vi "vision angle analysis.vi"(0 "left_x":dbl, 5 "right_x":dbl, 7 "top_y":dbl, 9 "bottom_y":dbl, 11 "gyro_angle_deg":dbl) -> (4 "gyro_heading_deg":dbl, 15 "distance":dbl)   [LabVIEW 2015]
panel:
  out "other distance":dbl
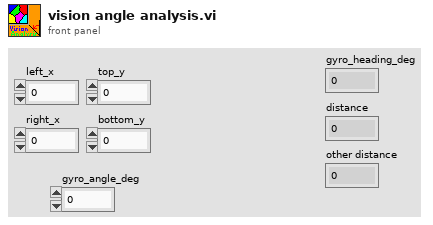
[diagram p1: front panel]
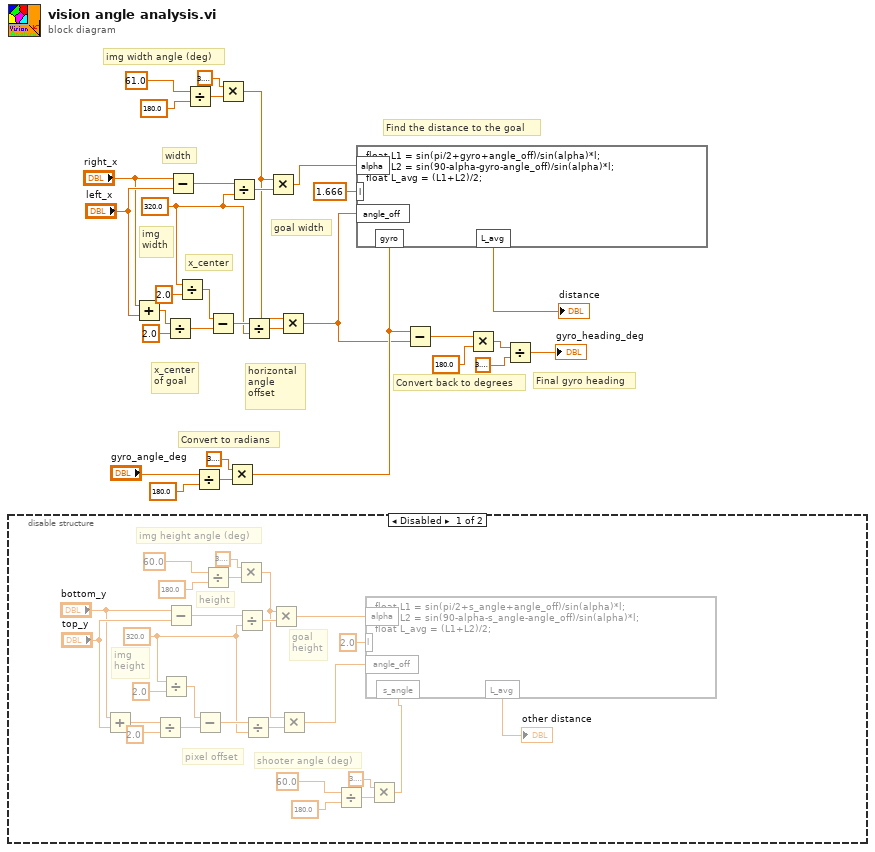
[diagram p0: block diagram]
diagram:
  w1 = 320.0 ("y")
  # "Find the distance to the goal"
  # "Convert back to degrees"
  # "Final gyro heading"
  # "horizontal \nangle \noffset"
  # "x_center"
  # "x_center\nof goal"
  # "Convert to radians"
  # "goal width"
  # "img width angle (deg)"
  # "img\nwidth"
  # "width"
  n1 = disable-structure shown="Disabled" {
    frame Disabled {
      w41 = 320.0 ("y")
      # "shooter angle (deg)"
      # "pixel offset"
      # "goal\nheight"
      # "img height angle (deg)"
      # "img\nheight"
      # "height"
      n2 = Add(x="bottom_y", y="top_y") -> (x+y=w46:dbl)
      n3 = Divide(x=w46, y=2.0) -> (x/y=w44:dbl)
      n4 = Divide(x=w41, y=2.0) -> (x/y=w43:dbl)
      n5 = Subtract(x="bottom_y", y="top_y") -> (x-y=w57:dbl)
      n6 = Subtract(x=w43, y=w44) -> (x-y=w42:dbl)
      n7 = Divide(x=60.0, y=180.0) -> (x/y=w54:dbl)
      n8 = Multiply(x=3.141592653589793, y=w54) -> (x*y=w39:dbl)
      n9 = Divide(x=w57, y=w41) -> (x/y=w56:dbl)
      n10 = Divide(x=w42, y=w41) -> (x/y=w40:dbl)
      n11 = Multiply(x=w39, y=w56) -> (x*y=w51:dbl)
      n12 = Multiply(x=w39, y=w40) -> (x*y=w38:dbl)
      n13 = Divide(x=60.0, y=180.0) -> (x/y=w36:dbl)
      n14 = Multiply(x=3.141592653589793, y=w36) -> (x*y=w33:dbl)
      n15 = formula code="float L1 = sin(pi/2+s_angle+angle_off)/sin(alpha)*l;\nfloat L2 = sin(90-alpha-s_angle-angle_off)/sin(alpha)*l;\nfloat L_avg = (L1+L2)/2;"("l"=2.0 ("input variable"), "alpha"=w51, "s_angle"=w33, "angle_off"=w38) -> ("L_avg"=→"other distance":dbl)
    }
    frame Enabled {
    }
  }
  n16 = Add(x="right_x", y="left_x") -> (x+y=w23:dbl)
  n17 = Divide(x=w23, y=2.0) -> (x/y=w19:dbl)
  n18 = Subtract(x="right_x", y="left_x") -> (x-y=w31:dbl)
  n19 = Divide(x=w1, y=2.0) -> (x/y=w3:dbl)
  n20 = Divide(x=61.0, y=180.0) -> (x/y=w7:dbl)
  n21 = Divide(x="gyro_angle_deg", y=180.0) -> (x/y=w25:dbl)
  n22 = Subtract(x=w3, y=w19) -> (x-y=w18:dbl)
  n23 = Multiply(x=3.141592653589793, y=w7) -> (x*y=w6:dbl)
  n24 = Multiply(x=3.141592653589793, y=w25) -> (x*y=w10:dbl)
  n25 = Divide(x=w31, y=w1) -> (x/y=w30:dbl)
  n26 = Divide(x=w18, y=w1) -> (x/y=w17:dbl)
  n27 = Multiply(x=w6, y=w30) -> (x*y=w29:dbl)
  n28 = Multiply(x=w6, y=w17) -> (x*y=w9:dbl)
  n29 = formula code="float L1 = sin(pi/2+gyro+angle_off)/sin(alpha)*l;\nfloat L2 = sin(90-alpha-gyro-angle_off)/sin(alpha)*l;\nfloat L_avg = (L1+L2)/2;"("l"=1.666 ("input variable"), "alpha"=w29, "gyro"=w10, "angle_off"=w9) -> ("L_avg"=→"distance":dbl)
  n30 = Subtract(x=w10, y=w9) -> (x-y=w11:dbl)
  n31 = Multiply(x=w11, y=180.0) -> (x*y=w14:dbl)
  n32 = Divide(x=w14, y=3.141592653589793) -> (x/y=→"gyro_heading_deg":dbl)
